vi "InitializeCapCamCaptureAndGraph.vi"(6 "Image mapping Array":T10[](array[typedef])=[{"Cam Cap Map Info"={"Cap Grid Info In"=[[{"Cap Type"=enum."Cap Form", "Scaling"=0.0, "Cap Num"=0, "center X"=0, "center Y"=0, "side length"=0}, {"Cap Type"=enum."Rail Gap Trigger", "Scaling"=1.0, "Cap Num"=299, "center X"=0, "center Y"=0, "side length"=0}, {"Cap Type"=enum."Cap Form", "Scaling"=0.0, "Cap Num"=0, "center X"=0, "center Y"=0, "side length"=0}, {"Cap Type"=enum."Cap Form", "Scaling"=0.0, "Cap Num"=0, "center X"=0, "center Y"=0, "side length"=0}, {"Cap Type"=enum."Cap Form", "Scaling"=0.0, "Cap Num"=0, "center X"=0, "center Y"=0, "side length"=0}, {"Cap Type"=enum."Cap Form", "Scaling"=0.0, "Cap Num"=0, "center X"=0, "center Y"=0, "side length"=0}, {"Cap Type"=enum."Cap Preform", "Scaling"=1.0, "Cap Num"=298, "center X"=0, "center Y"=0, "side length"=0}, {"Cap Type"=enum."Cap Form", "Scaling"=0.0, "Cap Num"=0, "center X"=0, "center Y"=0, "side length"=0}, {"Cap Type"=enum."Cap Form", "Scaling"=0.0, "Cap Num"=0, "center X"=0, "center Y"=0, "side length"=0}, {"Cap Type"=enum."Cap Form", "Scaling"=0.0, "Cap Num"=0, "center X"=0, "center Y"=0, "side length"=0}], [{"Cap Type"=enum."Cap Form", "Scaling"=0.0, "Cap Num"=0, "center X"=0, "center Y"=0, "side length"=0}, {"Cap Type"=enum."Cap Form", "Scaling"=0.0, "Cap Num"=0, "center X"=0, "center Y"=0, "side length"=0}, {"Cap Type"=enum."Cap Form", "Scaling"=0.0, "Cap Num"=0, "center X"=0, "center Y"=0, "side length"=0}, {"Cap Type"=enum."Cap Form", "Scaling"=0.0, "Cap Num"=0, "center X"=0, "center Y"=0, "side length"=0}, {"Cap Type"=enum."Cap Form", "Scaling"=0.0, "Cap Num"=0, "center X"=0, "center Y"=0, "side length"=0}, {"Cap Type"=enum."Cap Form", "Scaling"=0.0, "Cap Num"=0, "center X"=0, "center Y"=0, "side length"=0}, {"Cap Type"=enum."Cap Form", "Scaling"=0.0, "Cap Num"=0, "center X"=0, "center Y"=0, "side length"=0}, {"Cap Type"=enum."Cap Form", "Scaling"=0.0, "Cap Num"=0, "center X"=0, "center Y"=0, "side length"=0}, {"Cap Type"=enum."Cap Form", "Scaling"=0.0, "Cap Num"=0, "center X"=0, "center Y"=0, "side length"=0}, {"Cap Type"=enum."Cap Form", "Scaling"=0.0, "Cap Num"=0, "center X"=0, "center Y"=0, "side length"=0}], [{"Cap Type"=enum."Cap Form", "Scaling"=0.0, "Cap Num"=0, "center X"=0, "center Y"=0, "side length"=0}, {"Cap Type"=enum."Cap Form", "Scaling"=0.0, "Cap Num"=0, "center X"=0, "center Y"=0, "side length"=0}, {"Cap Type"=enum."Cap Form", "Scaling"=0.0, "Cap Num"=0, "center X"=0, "center Y"=0, "side length"=0}, {"Cap Type"=enum."Cap Form", "Scaling"=0.0, "Cap Num"=0, "center X"=0, "center Y"=0, "side length"=0}, {"Cap Type"=enum."Cap Form", "Scaling"=0.0, "Cap Num"=0, "center X"=0, "center Y"=0, "side length"=0}, {"Cap Type"=enum."Cap Form", "Scaling"=0.0, "Cap Num"=0, "center X"=0, "center Y"=0, "side length"=0}, {"Cap Type"=enum."Cap Form", "Scaling"=0.0, "Cap Num"=0, "center X"=0, "center Y"=0, "side length"=0}, {"Cap Type"=enum."Cap Form", "Scaling"=0.0, "Cap Num"=0, "center X"=0, "center Y"=0, "side length"=0}, {"Cap Type"=enum."Cap Form", "Scaling"=0.0, "Cap Num"=0, "center X"=0, "center Y"=0, "side length"=0}, {"Cap Type"=enum."Cap Form", "Scaling"=0.0, "Cap Num"=0, "center X"=0, "center Y"=0, "side length"=0}], [{"Cap Type"=enum."Cap Form", "Scaling"=0.0, "Cap Num"=0, "center X"=0, "center Y"=0, "side length"=0}, {"Cap Type"=enum."Cap Form", "Scaling"=0.0, "Cap Num"=0, "center X"=0, "center Y"=0, "side length"=0}, {"Cap Type"=enum."Cap Form", "Scaling"=0.0, "Cap Num"=0, "center X"=0, "center Y"=0, "side length"=0}, {"Cap Type"=enum."Cap Form", "Scaling"=0.0, "Cap Num"=0, "center X"=0, "center Y"=0, "side length"=0}, {"Cap Type"=enum."Cap Form", "Scaling"=0.0, "Cap Num"=0, "center X"=0, "center Y"=0, "side length"=0}, {"Cap Type"=enum."Cap Form", "Scaling"=0.0, "Cap Num"=0, "center X"=0, "center Y"=0, "side length"=0}, {"Cap Type"=enum."Cap Form", "Scaling"=0.0, "Cap Num"=0, "center X"=0, "center Y"=0, "side length"=0}, {"Cap Type"=enum."Cap Form", "Scaling"=0.0, "Cap Num"=0, "center X"=0, "center Y"=0, "side length"=0}, {"Cap Type"=enum."Cap Form", "Scaling"=0.0, "Cap Num"=0, "center X"=0, "center Y"=0, "side length"=0}, {"Cap Type"=enum."Cap Form", "Scaling"=0.0, "Cap Num"=0, "center X"=0, "center Y"=0, "side length"=0}], [{"Cap Type"=enum."Cap Form", "Scaling"=0.0, "Cap Num"=0, "center X"=0, "center Y"=0, "side length"=0}, {"Cap Type"=enum."Cap Form", "Scaling"=0.0, "Cap Num"=0, "center X"=0, "center Y"=0, "side length"=0}, {"Cap Type"=enum."Cap Form", "Scaling"=0.0, "Cap Num"=0, "center X"=0, "center Y"=0, "side length"=0}, {"Cap Type"=enum."Cap Form", "Scaling"=0.0, "Cap Num"=0, "center X"=0, "center Y"=0, "side length"=0}, {"Cap Type"=enum."Cap Form", "Scaling"=0.0, "Cap Num"=0, "center X"=0, "center Y"=0, "side length"=0}, {"Cap Type"=enum."Cap Form", "Scaling"=0.0, "Cap Num"=0, "center X"=0, "center Y"=0, "side length"=0}, {"Cap Type"=enum."Cap Form", "Scaling"=0.0, "Cap Num"=0, "center X"=0, "center Y"=0, "side length"=0}, {"Cap Type"=enum."Cap Form", "Scaling"=0.0, "Cap Num"=0, "center X"=0, "center Y"=0, "side length"=0}, {"Cap Type"=enum."Cap Form", "Scaling"=0.0, "Cap Num"=0, "center X"=0, "center Y"=0, "side length"=0}, {"Cap Type"=enum."Cap Form", "Scaling"=0.0, "Cap Num"=0, "center X"=0, "center Y"=0, "side length"=0}], [{"Cap Type"=enum."Cap Form", "Scaling"=1.0, "Cap Num"=340, "center X"=0, "center Y"=0, "side length"=0}, {"Cap Type"=enum."Cap Form", "Scaling"=1.0, "Cap Num"=341, "center X"=0, "center Y"=0, "side length"=0}, {"Cap Type"=enum."Cap Form", "Scaling"=1.0, "Cap Num"=342, "center X"=0, "center Y"=0, "side length"=0}, {"Cap Type"=enum."Cap Form", "Scaling"=1.0, "Cap Num"=343, "center X"=0, "center Y"=0, "side length"=0}, {"Cap Type"=enum."Cap Form", "Scaling"=1.0, "Cap Num"=344, "center X"=0, "center Y"=0, "side length"=0}, {"Cap Type"=enum."Cap Form", "Scaling"=1.0, "Cap Num"=345, "center X"=0, "center Y"=0, "side length"=0}, {"Cap Type"=enum."Cap Form", "Scaling"=1.0, "Cap Num"=346, "center X"=0, "center Y"=0, "side length"=0}, {"Cap Type"=enum."Cap Form", "Scaling"=1.0, "Cap Num"=347, "center X"=0, "center Y"=0, "side length"=0}, {"Cap Type"=enum."Cap Form", "Scaling"=0.0, "Cap Num"=0, "center X"=0, "center Y"=0, "side length"=0}, {"Cap Type"=enum."Cap Form", "Scaling"=0.0, "Cap Num"=0, "center X"=0, "center Y"=0, "side length"=0}], [{"Cap Type"=enum."Cap Form", "Scaling"=1.0, "Cap Num"=330, "center X"=0, "center Y"=0, "side length"=0}, {"Cap Type"=enum."Cap Form", "Scaling"=1.0, "Cap Num"=331, "center X"=0, "center Y"=0, "side length"=0}, {"Cap Type"=enum."Cap Form", "Scaling"=1.0, "Cap Num"=332, "center X"=0, "center Y"=0, "side length"=0}, {"Cap Type"=enum."Cap Form", "Scaling"=1.0, "Cap Num"=333, "center X"=0, "center Y"=0, "side length"=0}, {"Cap Type"=enum."Cap Form", "Scaling"=1.0, "Cap Num"=334, "center X"=0, "center Y"=0, "side length"=0}, {"Cap Type"=enum."Cap Form", "Scaling"=1.0, "Cap Num"=335, "center X"=0, "center Y"=0, "side length"=0}, {"Cap Type"=enum."Cap Form", "Scaling"=1.0, "Cap Num"=336, "center X"=0, "center Y"=0, "side length"=0}, {"Cap Type"=enum."Cap Form", "Scaling"=1.0, "Cap Num"=337, "center X"=0, "center Y"=0, "side length"=0}, {"Cap Type"=enum."Cap Form", "Scaling"=1.0, "Cap Num"=338, "center X"=0, "center Y"=0, "side length"=0}, {"Cap Type"=enum."Cap Form", "Scaling"=1.0, "Cap Num"=339, "center X"=0, "center Y"=0, "side length"=0}], [{"Cap Type"=enum."Cap Form", "Scaling"=1.0, "Cap Num"=320, "center X"=0, "center Y"=0, "side length"=0}, {"Cap Type"=enum."Cap Form", "Scaling"=1.0, "Cap Num"=321, "center X"=0, "center Y"=0, "side length"=0}, {"Cap Type"=enum."Cap Form", "Scaling"=1.0, "Cap Num"=322, "center X"=0, "center Y"=0, "side length"=0}, {"Cap Type"=enum."Cap Form", "Scaling"=1.0, "Cap Num"=323, "center X"=0, "center Y"=0, "side length"=0}, {"Cap Type"=enum."Cap Form", "Scaling"=1.0, "Cap Num"=324, "center X"=0, "center Y"=0, "side length"=0}, {"Cap Type"=enum."Cap Form", "Scaling"=1.0, "Cap Num"=325, "center X"=0, "center Y"=0, "side length"=0}, {"Cap Type"=enum."Cap Form", "Scaling"=1.0, "Cap Num"=326, "center X"=0, "center Y"=0, "side length"=0}, {"Cap Type"=enum."Cap Form", "Scaling"=1.0, "Cap Num"=327, "center X"=0, "center Y"=0, "side length"=0}, {"Cap Type"=enum."Cap Form", "Scaling"=1.0, "Cap Num"=328, "center X"=0, "center Y"=0, "side length"=0}, {"Cap Type"=enum."Cap Form", "Scaling"=1.0, "Cap Num"=329, "center X"=0, "center Y"=0, "side length"=0}], [{"Cap Type"=enum."Cap Form", "Scaling"=1.0, "Cap Num"=310, "center X"=0, "center Y"=0, "side length"=0}, {"Cap Type"=enum."Cap Form", "Scaling"=1.0, "Cap Num"=311, "center X"=0, "center Y"=0, "side length"=0}, {"Cap Type"=enum."Cap Form", "Scaling"=1.0, "Cap Num"=312, "center X"=0, "center Y"=0, "side length"=0}, {"Cap Type"=enum."Cap Form", "Scaling"=1.0, "Cap Num"=313, "center X"=0, "center Y"=0, "side length"=0}, {"Cap Type"=enum."Cap Form", "Scaling"=1.0, "Cap Num"=314, "center X"=0, "center Y"=0, "side length"=0}, {"Cap Type"=enum."Cap Form", "Scaling"=1.0, "Cap Num"=315, "center X"=0, "center Y"=0, "side length"=0}, {"Cap Type"=enum."Cap Form", "Scaling"=1.0, "Cap Num"=316, "center X"=0, "center Y"=0, "side length"=0}, {"Cap Type"=enum."Cap Form", "Scaling"=1.0, "Cap Num"=317, "center X"=0, "center Y"=0, "side length"=0}, {"Cap Type"=enum."Cap Form", "Scaling"=1.0, "Cap Num"=318, "center X"=0, "center Y"=0, "side length"=0}, {"Cap Type"=enum."Cap Form", "Scaling"=1.0, "Cap Num"=319, "center X"=0, "center Y"=0, "side length"=0}], [{"Cap Type"=enum."Cap Form", "Scaling"=1.0, "Cap Num"=300, "center X"=0, "center Y"=0, "side length"=0}, {"Cap Type"=enum."Cap Form", "Scaling"=1.0, "Cap Num"=301, "center X"=0, "center Y"=0, "side length"=0}, {"Cap Type"=enum."Cap Form", "Scaling"=1.0, "Cap Num"=302, "center X"=0, "center Y"=0, "side length"=0}, {"Cap Type"=enum."Cap Form", "Scaling"=1.0, "Cap Num"=303, "center X"=0, "center Y"=0, "side length"=0}, {"Cap Type"=enum."Cap Form", "Scaling"=1.0, "Cap Num"=304, "center X"=0, "center Y"=0, "side length"=0}, {"Cap Type"=enum."Cap Form", "Scaling"=1.0, "Cap Num"=305, "center X"=0, "center Y"=0, "side length"=0}, {"Cap Type"=enum."Cap Form", "Scaling"=1.0, "Cap Num"=306, "center X"=0, "center Y"=0, "side length"=0}, {"Cap Type"=enum."Cap Form", "Scaling"=1.0, "Cap Num"=307, "center X"=0, "center Y"=0, "side length"=0}, {"Cap Type"=enum."Cap Form", "Scaling"=1.0, "Cap Num"=308, "center X"=0, "center Y"=0, "side length"=0}, {"Cap Type"=enum."Cap Form", "Scaling"=1.0, "Cap Num"=309, "center X"=0, "center Y"=0, "side length"=0}]], "Solid Colour Threshold"=1}, "DAQ Image Name"="CapVoltCam"}, {"Cam Cap Map Info"={"Cap Grid Info In"=[[{"Cap Type"=enum."Cap Peaking", "Scaling"=1.0, "Cap Num"=378, "center X"=0, "center Y"=0, "side length"=0}, {"Cap Type"=enum."Cap Peaking", "Scaling"=1.0, "Cap Num"=379, "center X"=0, "center Y"=0, "side length"=0}, {"Cap Type"=enum."Cap Peaking", "Scaling"=1.0, "Cap Num"=384, "center X"=0, "center Y"=0, "side length"=0}, {"Cap Type"=enum."Cap Peaking", "Scaling"=1.0, "Cap Num"=385, "center X"=0, "center Y"=0, "side length"=0}, {"Cap Type"=enum."Cap Peaking", "Scaling"=1.0, "Cap Num"=390, "center X"=0, "center Y"=0, "side length"=0}, {"Cap Type"=enum."Cap Peaking", "Scaling"=1.0, "Cap Num"=391, "center X"=0, "center Y"=0, "side length"=0}, {"Cap Type"=enum."Cap Peaking", "Scaling"=0.0, "Cap Num"=0, "center X"=0, "center Y"=0, "side length"=0}, {"Cap Type"=enum."Cap Peaking", "Scaling"=0.0, "Cap Num"=0, "center X"=0, "center Y"=0, "side length"=0}, {"Cap Type"=enum."Cap Peaking", "Scaling"=0.0, "Cap Num"=0, "center X"=0, "center Y"=0, "side length"=0}, {"Cap Type"=enum."Cap Peaking", "Scaling"=0.0, "Cap Num"=0, "center X"=0, "center Y"=0, "side length"=0}], [{"Cap Type"=enum."Cap Peaking", "Scaling"=1.0, "Cap Num"=348, "center X"=0, "center Y"=0, "side length"=0}, {"Cap Type"=enum."Cap Peaking", "Scaling"=1.0, "Cap Num"=349, "center X"=0, "center Y"=0, "side length"=0}, {"Cap Type"=enum."Cap Peaking", "Scaling"=1.0, "Cap Num"=354, "center X"=0, "center Y"=0, "side length"=0}, {"Cap Type"=enum."Cap Peaking", "Scaling"=1.0, "Cap Num"=355, "center X"=0, "center Y"=0, "side length"=0}, {"Cap Type"=enum."Cap Peaking", "Scaling"=1.0, "Cap Num"=360, "center X"=0, "center Y"=0, "side length"=0}, {"Cap Type"=enum."Cap Peaking", "Scaling"=1.0, "Cap Num"=361, "center X"=0, "center Y"=0, "side length"=0}, {"Cap Type"=enum."Cap Peaking", "Scaling"=1.0, "Cap Num"=366, "center X"=0, "center Y"=0, "side length"=0}, {"Cap Type"=enum."Cap Peaking", "Scaling"=1.0, "Cap Num"=367, "center X"=0, "center Y"=0, "side length"=0}, {"Cap Type"=enum."Cap Peaking", "Scaling"=1.0, "Cap Num"=372, "center X"=0, "center Y"=0, "side length"=0}, {"Cap Type"=enum."Cap Peaking", "Scaling"=1.0, "Cap Num"=373, "center X"=0, "center Y"=0, "side length"=0}], [{"Cap Type"=enum."Cap Peaking", "Scaling"=0.0, "Cap Num"=0, "center X"=0, "center Y"=0, "side length"=0}, {"Cap Type"=enum."Cap Peaking", "Scaling"=0.0, "Cap Num"=0, "center X"=0, "center Y"=0, "side length"=0}, {"Cap Type"=enum."Cap Peaking", "Scaling"=0.0, "Cap Num"=0, "center X"=0, "center Y"=0, "side length"=0}, {"Cap Type"=enum."Cap Peaking", "Scaling"=0.0, "Cap Num"=0, "center X"=0, "center Y"=0, "side length"=0}, {"Cap Type"=enum."Cap Peaking", "Scaling"=0.0, "Cap Num"=0, "center X"=0, "center Y"=0, "side length"=0}, {"Cap Type"=enum."Cap Peaking", "Scaling"=0.0, "Cap Num"=0, "center X"=0, "center Y"=0, "side length"=0}, {"Cap Type"=enum."Cap Peaking", "Scaling"=0.0, "Cap Num"=0, "center X"=0, "center Y"=0, "side length"=0}, {"Cap Type"=enum."Cap Peaking", "Scaling"=0.0, "Cap Num"=0, "center X"=0, "center Y"=0, "side length"=0}, {"Cap Type"=enum."Cap Peaking", "Scaling"=0.0, "Cap Num"=0, "center X"=0, "center Y"=0, "side length"=0}, {"Cap Type"=enum."Cap Peaking", "Scaling"=0.0, "Cap Num"=0, "center X"=0, "center Y"=0, "side length"=0}], [{"Cap Type"=enum."Cap Peaking", "Scaling"=0.0, "Cap Num"=0, "center X"=0, "center Y"=0, "side length"=0}, {"Cap Type"=enum."Cap Peaking", "Scaling"=0.0, "Cap Num"=0, "center X"=0, "center Y"=0, "side length"=0}, {"Cap Type"=enum."Cap Peaking", "Scaling"=0.0, "Cap Num"=0, "center X"=0, "center Y"=0, "side length"=0}, {"Cap Type"=enum."Cap Peaking", "Scaling"=0.0, "Cap Num"=0, "center X"=0, "center Y"=0, "side length"=0}, {"Cap Type"=enum."Cap Peaking", "Scaling"=0.0, "Cap Num"=0, "center X"=0, "center Y"=0, "side length"=0}, {"Cap Type"=enum."Cap Peaking", "Scaling"=0.0, "Cap Num"=0, "center X"=0, "center Y"=0, "side length"=0}, {"Cap Type"=enum."Cap Peaking", "Scaling"=0.0, "Cap Num"=0, "center X"=0, "center Y"=0, "side length"=0}, {"Cap Type"=enum."Cap Peaking", "Scaling"=0.0, "Cap Num"=0, "center X"=0, "center Y"=0, "side length"=0}, {"Cap Type"=enum."Cap Peaking", "Scaling"=0.0, "Cap Num"=0, "center X"=0, "center Y"=0, "side length"=0}, {"Cap Type"=enum."Cap Peaking", "Scaling"=0.0, "Cap Num"=0, "center X"=0, "center Y"=0, "side length"=0}], [{"Cap Type"=enum."Cap Peaking", "Scaling"=0.0, "Cap Num"=0, "center X"=0, "center Y"=0, "side length"=0}, {"Cap Type"=enum."Cap Peaking", "Scaling"=0.0, "Cap Num"=0, "center X"=0, "center Y"=0, "side length"=0}, {"Cap Type"=enum."Cap Peaking", "Scaling"=0.0, "Cap Num"=0, "center X"=0, "center Y"=0, "side length"=0}, {"Cap Type"=enum."Cap Peaking", "Scaling"=0.0, "Cap Num"=0, "center X"=0, "center Y"=0, "side length"=0}, {"Cap Type"=enum."Cap Peaking", "Scaling"=0.0, "Cap Num"=0, "center X"=0, "center Y"=0, "side length"=0}, {"Cap Type"=enum."Cap Peaking", "Scaling"=0.0, "Cap Num"=0, "center X"=0, "center Y"=0, "side length"=0}, {"Cap Type"=enum."Cap Peaking", "Scaling"=0.0, "Cap Num"=0, "center X"=0, "center Y"=0, "side length"=0}, {"Cap Type"=enum."Cap Peaking", "Scaling"=0.0, "Cap Num"=0, "center X"=0, "center Y"=0, "side length"=0}, {"Cap Type"=enum."Cap Peaking", "Scaling"=0.0, "Cap Num"=0, "center X"=0, "center Y"=0, "side length"=0}, {"Cap Type"=enum."Cap Peaking", "Scaling"=0.0, "Cap Num"=0, "center X"=0, "center Y"=0, "side length"=0}], [{"Cap Type"=enum."Cap Peaking", "Scaling"=0.0, "Cap Num"=0, "center X"=0, "center Y"=0, "side length"=0}, {"Cap Type"=enum."Cap Peaking", "Scaling"=0.0, "Cap Num"=0, "center X"=0, "center Y"=0, "side length"=0}, {"Cap Type"=enum."Cap Peaking", "Scaling"=0.0, "Cap Num"=0, "center X"=0, "center Y"=0, "side length"=0}, {"Cap Type"=enum."Cap Peaking", "Scaling"=0.0, "Cap Num"=0, "center X"=0, "center Y"=0, "side length"=0}, {"Cap Type"=enum."Cap Peaking", "Scaling"=0.0, "Cap Num"=0, "center X"=0, "center Y"=0, "side length"=0}, {"Cap Type"=enum."Cap Peaking", "Scaling"=0.0, "Cap Num"=0, "center X"=0, "center Y"=0, "side length"=0}, {"Cap Type"=enum."Cap Peaking", "Scaling"=0.0, "Cap Num"=0, "center X"=0, "center Y"=0, "side length"=0}, {"Cap Type"=enum."Cap Peaking", "Scaling"=0.0, "Cap Num"=0, "center X"=0, "center Y"=0, "side length"=0}, {"Cap Type"=enum."Cap Peaking", "Scaling"=0.0, "Cap Num"=0, "center X"=0, "center Y"=0, "side length"=0}, {"Cap Type"=enum."Cap Peaking", "Scaling"=0.0, "Cap Num"=0, "center X"=0, "center Y"=0, "side length"=0}], [{"Cap Type"=enum."Cap Peaking", "Scaling"=0.0, "Cap Num"=0, "center X"=0, "center Y"=0, "side length"=0}, {"Cap Type"=enum."Cap Peaking", "Scaling"=0.0, "Cap Num"=0, "center X"=0, "center Y"=0, "side length"=0}, {"Cap Type"=enum."Cap Peaking", "Scaling"=0.0, "Cap Num"=0, "center X"=0, "center Y"=0, "side length"=0}, {"Cap Type"=enum."Cap Peaking", "Scaling"=0.0, "Cap Num"=0, "center X"=0, "center Y"=0, "side length"=0}, {"Cap Type"=enum."Cap Peaking", "Scaling"=0.0, "Cap Num"=0, "center X"=0, "center Y"=0, "side length"=0}, {"Cap Type"=enum."Cap Peaking", "Scaling"=0.0, "Cap Num"=0, "center X"=0, "center Y"=0, "side length"=0}, {"Cap Type"=enum."Cap Peaking", "Scaling"=0.0, "Cap Num"=0, "center X"=0, "center Y"=0, "side length"=0}, {"Cap Type"=enum."Cap Peaking", "Scaling"=0.0, "Cap Num"=0, "center X"=0, "center Y"=0, "side length"=0}, {"Cap Type"=enum."Cap Peaking", "Scaling"=0.0, "Cap Num"=0, "center X"=0, "center Y"=0, "side length"=0}, {"Cap Type"=enum."Cap Peaking", "Scaling"=0.0, "Cap Num"=0, "center X"=0, "center Y"=0, "side length"=0}], [{"Cap Type"=enum."Cap Peaking", "Scaling"=0.0, "Cap Num"=0, "center X"=0, "center Y"=0, "side length"=0}, {"Cap Type"=enum."Cap Peaking", "Scaling"=0.0, "Cap Num"=0, "center X"=0, "center Y"=0, "side length"=0}, {"Cap Type"=enum."Cap Peaking", "Scaling"=0.0, "Cap Num"=0, "center X"=0, "center Y"=0, "side length"=0}, {"Cap Type"=enum."Cap Peaking", "Scaling"=0.0, "Cap Num"=0, "center X"=0, "center Y"=0, "side length"=0}, {"Cap Type"=enum."Cap Peaking", "Scaling"=0.0, "Cap Num"=0, "center X"=0, "center Y"=0, "side length"=0}, {"Cap Type"=enum."Cap Peaking", "Scaling"=0.0, "Cap Num"=0, "center X"=0, "center Y"=0, "side length"=0}, {"Cap Type"=enum."Cap Peaking", "Scaling"=0.0, "Cap Num"=0, "center X"=0, "center Y"=0, "side length"=0}, {"Cap Type"=enum."Cap Peaking", "Scaling"=0.0, "Cap Num"=0, "center X"=0, "center Y"=0, "side length"=0}, {"Cap Type"=enum."Cap Peaking", "Scaling"=0.0, "Cap Num"=0, "center X"=0, "center Y"=0, "side length"=0}, {"Cap Type"=enum."Cap Peaking", "Scaling"=0.0, "Cap Num"=0, "center X"=0, "center Y"=0, "side length"=0}], [{"Cap Type"=enum."Cap Peaking", "Scaling"=0.0, "Cap Num"=0, "center X"=0, "center Y"=0, "side length"=0}, {"Cap Type"=enum."Cap Peaking", "Scaling"=0.0, "Cap Num"=0, "center X"=0, "center Y"=0, "side length"=0}, {"Cap Type"=enum."Cap Peaking", "Scaling"=0.0, "Cap Num"=0, "center X"=0, "center Y"=0, "side length"=0}, {"Cap Type"=enum."Cap Peaking", "Scaling"=0.0, "Cap Num"=0, "center X"=0, "center Y"=0, "side length"=0}, {"Cap Type"=enum."Cap Peaking", "Scaling"=0.0, "Cap Num"=0, "center X"=0, "center Y"=0, "side length"=0}, {"Cap Type"=enum."Cap Peaking", "Scaling"=0.0, "Cap Num"=0, "center X"=0, "center Y"=0, "side length"=0}, {"Cap Type"=enum."Cap Peaking", "Scaling"=0.0, "Cap Num"=0, "center X"=0, "center Y"=0, "side length"=0}, {"Cap Type"=enum."Cap Peaking", "Scaling"=0.0, "Cap Num"=0, "center X"=0, "center Y"=0, "side length"=0}, {"Cap Type"=enum."Cap Peaking", "Scaling"=0.0, "Cap Num"=0, "center X"=0, "center Y"=0, "side length"=0}, {"Cap Type"=enum."Cap Peaking", "Scaling"=0.0, "Cap Num"=0, "center X"=0, "center Y"=0, "side length"=0}], [{"Cap Type"=enum."Cap Peaking", "Scaling"=0.0, "Cap Num"=0, "center X"=0, "center Y"=0, "side length"=0}, {"Cap Type"=enum."Cap Peaking", "Scaling"=0.0, "Cap Num"=0, "center X"=0, "center Y"=0, "side length"=0}, {"Cap Type"=enum."Cap Peaking", "Scaling"=0.0, "Cap Num"=0, "center X"=0, "center Y"=0, "side length"=0}, {"Cap Type"=enum."Cap Peaking", "Scaling"=0.0, "Cap Num"=0, "center X"=0, "center Y"=0, "side length"=0}, {"Cap Type"=enum."Cap Peaking", "Scaling"=0.0, "Cap Num"=0, "center X"=0, "center Y"=0, "side length"=0}, {"Cap Type"=enum."Cap Peaking", "Scaling"=0.0, "Cap Num"=0, "center X"=0, "center Y"=0, "side length"=0}, {"Cap Type"=enum."Cap Peaking", "Scaling"=0.0, "Cap Num"=0, "center X"=0, "center Y"=0, "side length"=0}, {"Cap Type"=enum."Cap Peaking", "Scaling"=0.0, "Cap Num"=0, "center X"=0, "center Y"=0, "side length"=0}, {"Cap Type"=enum."Cap Peaking", "Scaling"=0.0, "Cap Num"=0, "center X"=0, "center Y"=0, "side length"=0}, {"Cap Type"=enum."Cap Peaking", "Scaling"=0.0, "Cap Num"=0, "center X"=0, "center Y"=0, "side length"=0}]], "Solid Colour Threshold"=1}, "DAQ Image Name"="CapCam2"}], 7 "Polling Camera Objects":T5[](array[typedef])=[{"DAQ Image"={"DAQ Image Name"="CapVoltCam", "Device Functional"=TRUE, "Channel Enabled"=TRUE, "Trigger Name"="", "Image Object"=refnum, "Camera Session"="CapVoltCam", "Time Stamp"=3627072022.67675}, "Image Configuration Cluster"={"DAQ Image Name"="Cam4Pic", "Serial Number"=207552104335, "Exposure (us)"=0.0, "Trigger Delay (us)"=0.0, "Raw Gain"=0.0, "Exposure Max (us)"=0.0, "Exposure Min (us)"=0.0, "Trigger Delay Max (us)"=0.0, "Trigger Delay Min (us)"=0.0, "Raw Gain Max"=0.0, "Raw Gain Min"=0.0, "Acquisition Mode"=0, "Trigger Mode"=0, "Trigger Source"=0, "Pixel Format"=0, "Resends Enabled"=0, "Max Test Packet Retries"=0, "Test Packet Timeout"=0, "Missing Packet Timeout"=0, "New Packet Timeout"=0, "Resend Response Timeout"=0}, "Minimum Time Between Frames (s)"=0.02, "error out"={"status"=FALSE, "code"=0, "source"=""}, "Required"=TRUE}, {"DAQ Image"={"DAQ Image Name"="CapCam2", "Device Functional"=TRUE, "Channel Enabled"=TRUE, "Trigger Name"="", "Image Object"=refnum, "Camera Session"="CapCam2", "Time Stamp"=3627072022.6897507}, "Image Configuration Cluster"={"DAQ Image Name"="Cam2Pic", "Serial Number"=207552146538, "Exposure (us)"=0.0, "Trigger Delay (us)"=0.0, "Raw Gain"=0.0, "Exposure Max (us)"=0.0, "Exposure Min (us)"=0.0, "Trigger Delay Max (us)"=0.0, "Trigger Delay Min (us)"=0.0, "Raw Gain Max"=0.0, "Raw Gain Min"=0.0, "Acquisition Mode"=0, "Trigger Mode"=0, "Trigger Source"=0, "Pixel Format"=0, "Resends Enabled"=0, "Max Test Packet Retries"=0, "Test Packet Timeout"=0, "Missing Packet Timeout"=0, "New Packet Timeout"=0, "Resend Response Timeout"=0}, "Minimum Time Between Frames (s)"=0.02, "error out"={"status"=FALSE, "code"=0, "source"=""}, "Required"=TRUE}], 8 "Graph Refnum In":refnum<vi>) -> (0 "Error Array":errorcluster[](array[cluster]), 1 "Initial Collection":T1[](array[typedef]), 2 "Initial Base Time":dbl, 3 "All Required Cams Working":bool, 4 "Initialized Polling Cameras":T5[](array[typedef]), 5 "Graph Refnum Out":refnum<vi>)   [LabVIEW 2016]
uses:
  Camera Controls/PollingCamera_HAL.ctl
  HardwareInterfaceLayer/ImageIn.ctl
  <vilib>/vision/Image Controls.llb/IMAQ Image.ctl
  <vilib>/userdefined/High Color/IMAQdx.ctl
  HardwareInterfaceLayer/ImageInConfig.ctl
  Camera Controls/ImageToGridMapping.ctl
  Camera Controls/CamCapMapInfo.ctl
  Camera Controls/CapElectrodeInfo.ctl
  Camera Controls/CapElectrodeChoices.ctl
  Camera Controls/CapTotalInfoAndDataArrayCluster.ctl
  Camera Controls/DataPointCluster.ctl
panel:
  out "Cap Voltage Graph":cluster{cluster{"Time":dbl, "data":dbl}[]}[](graph)
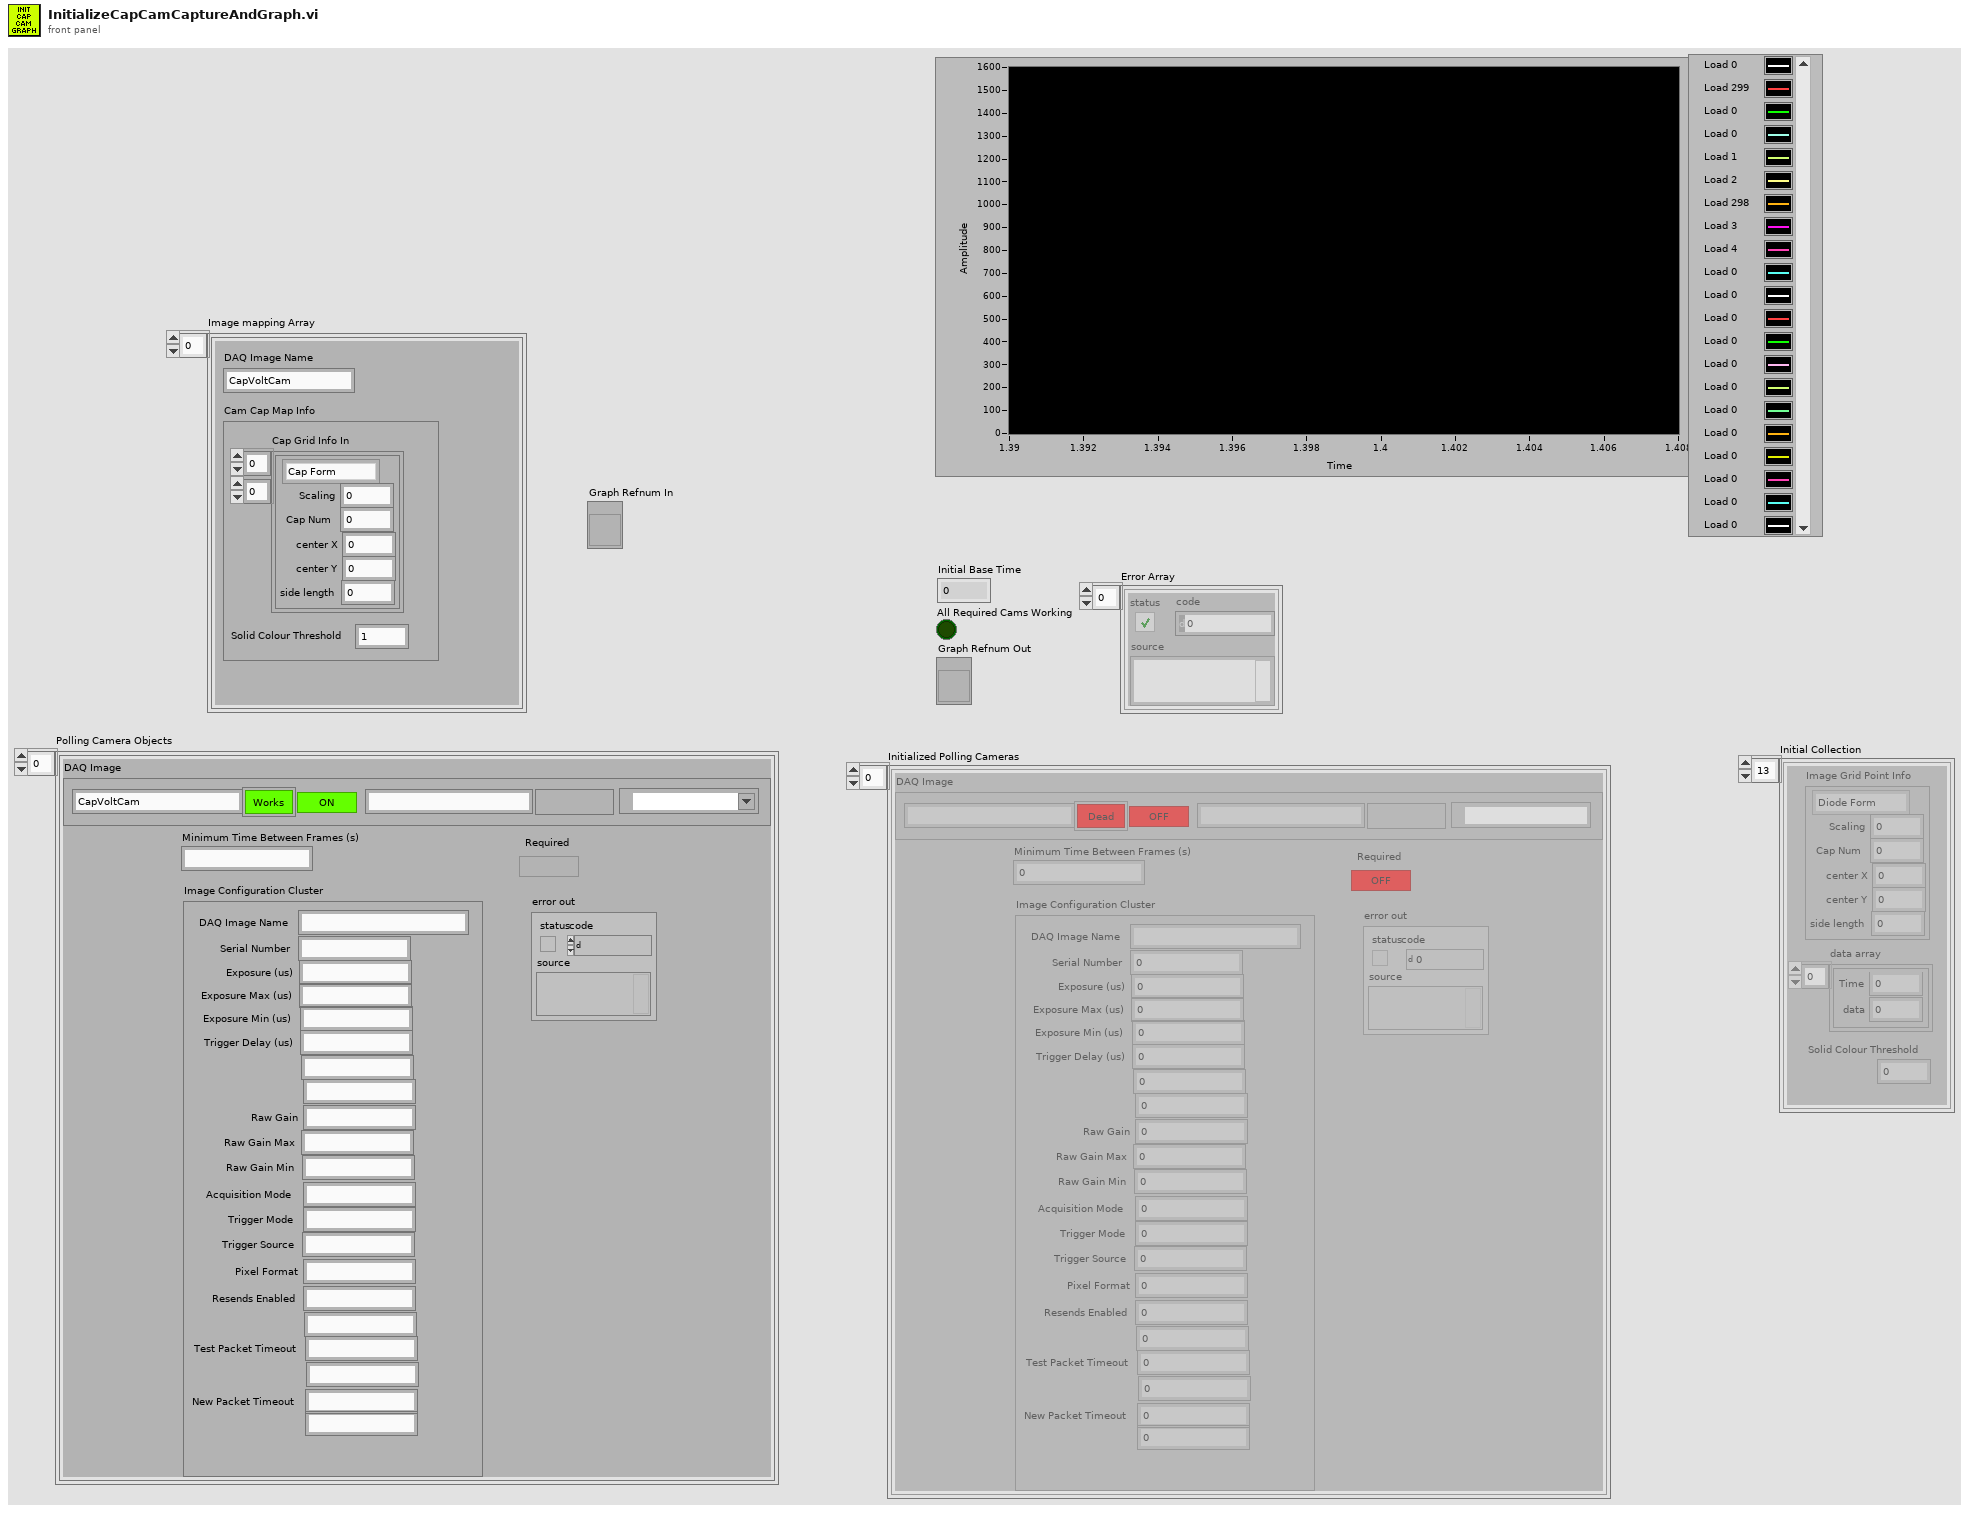
[diagram p1: front panel]
types:
  T1 = typedef "CapTotalInfoAndDataArrayCluster.ctl" = cluster{"Image Grid Point Info":T2, "data array":T4[], "Solid Colour Threshold":i32}
  T2 = typedef "CapElectrodeInfo.ctl" = cluster{"Cap Type":T3, "Scaling":dbl, "Cap Num":u32, "center X":u32, "center Y":u32, "side length":u32}
  T3 = typedef "CapElectrodeChoices.ctl" = enum16{"Diode Form", "Diode Preform", "Diode Pretor", "Diode Peaking", "Diode Sustain", "Diode Post Tor", "Cap Form", "Cap Preform", "Cap Pretor", "Cap Peaking", "Cap Sustain", "Cap Post Tor", "Rail Gap Trigger"}
  T4 = typedef "DataPointCluster.ctl" = cluster{"Time":dbl, "data":dbl}
  T5 = typedef "PollingCamera_HAL.ctl" = cluster{"DAQ Image":T6, "Image Configuration Cluster":T9, "Minimum Time Between Frames (s)":dbl, "error out":errorcluster, "Required":bool}
  T6 = typedef "ImageIn.ctl" = cluster{"DAQ Image Name":string, "Device Functional":bool, "Channel Enabled":bool, "Trigger Name":string, "Image Object":T7, "Camera Session":T8, "Time Stamp":dbl}
  T7 = typedef "IMAQ Image.ctl" = refnum<image>
  T8 = typedef "IMAQdx.ctl" = refnum<k21>
  T9 = typedef "ImageInConfig.ctl" = cluster{"DAQ Image Name":string, "Serial Number":u64, "Exposure (us)":dbl, "Trigger Delay (us)":dbl, "Raw Gain":dbl, "Exposure Max (us)":dbl, "Exposure Min (us)":dbl, "Trigger Delay Max (us)":dbl, "Trigger Delay Min (us)":dbl, "Raw Gain Max":dbl, "Raw Gain Min":dbl, "Acquisition Mode":u32, "Trigger Mode":u32, "Trigger Source":u32, "Pixel Format":u32, "Resends Enabled":u32, "Max Test Packet Retries":u32, "Test Packet Timeout":u32, "Missing Packet Timeout":u32, "New Packet Timeout":u32, "Resend Response Timeout":u32}
  T10 = typedef "ImageToGridMapping.ctl" = cluster{"Cam Cap Map Info":T11, "DAQ Image Name":string}
  T11 = typedef "CamCapMapInfo.ctl" = cluster{"Cap Grid Info In":T2[][], "Solid Colour Threshold":i32}
  T12 = typedef "CapTotalInfoAndDataCluster.ctl" = cluster{"Image Grid Point Info":T2, "Solid Colour Threshold":i32, "data cluster":T4}
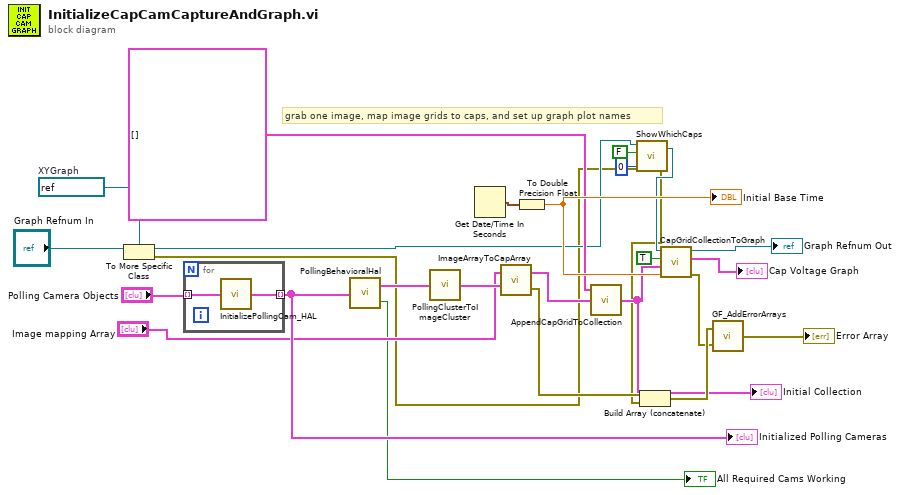
[diagram p0: block diagram]
diagram:
  w25 = refnum<vi> refnum  # XYGraph
  # "grab one image, map image grids to caps, and set up graph plot names"
  n1 = To More Specific Class(target class=w25, reference="Graph Refnum In") -> (specific class reference=w5:refnum<vi>, error out=w3:errorcluster)  [unwired: 1 in]
  n2 = for {
    tunnel: "Polling Camera Objects" -> [w28] mode=indexing
    tunnel: [w27] -> w23 mode=indexing
    n3 = call "InitializePollingCam_HAL.vi"("Polling Snap Camera In"=w28) -> ("Polling Snap Camera Out"=w27:T5)
  }
  "Initialized Polling Cameras" <- w23
  n4 = call "PollingBehavioralHal.vi"("Polling Camera In"=w23) -> ("Polling Camera Out"=w22:T5[], "All Required Cams Working"=→"All Required Cams Working":bool)
  n5 = call "PollingClusterToImageCluster.vi"("Polling Clusters In"=w22) -> ("Image Clusters Out"=w21:T6[])
  n6 = Get Date/Time In Seconds() -> (seconds since 1Jan1904=w19:timestamp)
  n7 = call "ImageArrayToCapArray.vi"("Images Array"=w21, "Image mapping Array"="Image mapping Array") -> ("Error Array"=w16:errorcluster[], "Cap Grid Info Array Out"=w7:T12[])
  n8 = To Double Precision Float(number=w19) -> (double precision float=w18:dbl)
  "Initial Base Time" <- w18
  n9 = call "AppendCapGridToCollection.vi"("Cap Grid Info Array"=w7, "Array of Caps in Grids In"=T1[] []) -> ("Array of Caps in Grids Out"=w9:T1[])  [unwired: 1 in]
  "Initial Collection" <- w9
  n10 = call "ShowWhichCaps.vi"("error in (no error)"=w3, "Cap Number To Show"=u32 0, "Only Show One Trace"=FALSE, "XYGraph Refnum In"=w5) -> ("error out"=w2:errorcluster, "XYGraph Refnum Out"=w4:refnum<vi>)
  n11 = Build Array (concatenate)(w16, w2) -> (w14:errorcluster[])
  n12 = call "CapGridCollectionToGraph.vi"("Base Time"=w18, "Cap Grid Collection"=w9, "Update Plot Attributes"=TRUE, "Graph Refnum In"=w4) -> ("Error Array"=w13:errorcluster[], "Cap Voltage Graph"=→"Cap Voltage Graph":cluster{cluster{"Time":dbl, "data":dbl}[]}[], "Graph Refnum Out"=→"Graph Refnum Out":refnum<vi>)  [unwired: 1 in, 1 out]
  n13 = call "GF_AddErrorArrays.vi"("Error Array To Add In"=w13, "Error Array In"=w14) -> ("Error Array Out"=→"Error Array":errorcluster[])
